vi "TaborBurst.vi"(0 "Input Cluster":T1={"Cycles"=0, "Therapy frequency (MHz)"=0.0, "Therapy amplitude (mV)"=50.0} {"Therapy amplitude (mV)" min=50.0 max=2000.0 format="%.2f"; "Therapy frequency (MHz)" format="%.2f"}, 1 "instrument in":refnum<k15>, 3 "error in (no error)":errorcluster) -> (5 "instrument out":refnum<k15>, 8 "error out":errorcluster)   [LabVIEW 2022 SP3]
uses:
  Pulsers/PulserGlobals.vi
panel:
  # "Set up to work with HP33120A. It is used as a burst source with\neither a gated burst or a fixed number of cycels"
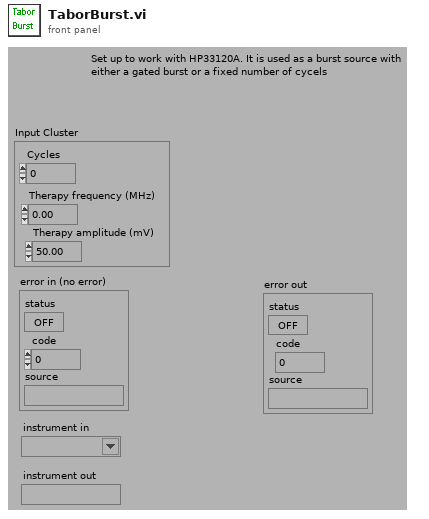
[diagram p1: front panel]
types:
  T1 = cluster{"Cycles":i32, "Therapy frequency (MHz)":dbl, "Therapy amplitude (mV)":dbl}
  T2 = cluster{"Therapy frequency (MHz)":dbl, "Therapy amplitude (mV)":dbl, "time therapy on (s)":dbl, "Therapy Delay (ms) ":dbl, "Time (s)":dbl}
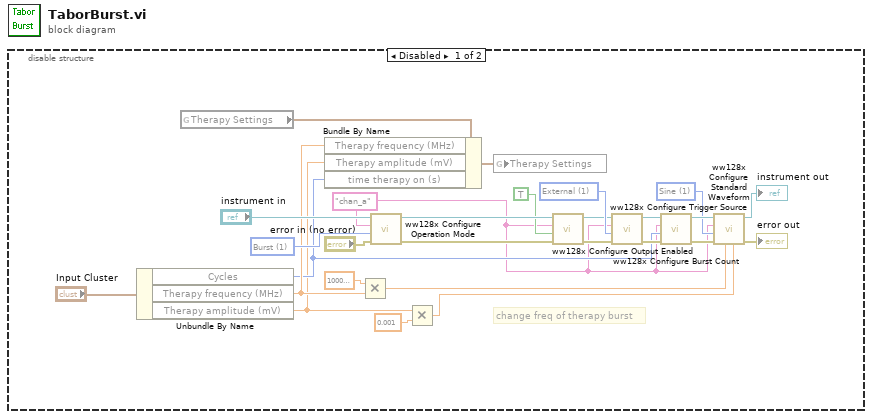
[diagram p0: block diagram]
diagram:
  n1 = disable-structure shown="Disabled" {
    frame Disabled {
      w1 = "chan_a" ("channel name (\"CHAN_A\")")
      w11 = 1 items=["External"=1, "Internal"=3, "Software Trigger"=2] ("source")
      w16 = 1 items=["Continuous"=0, "Burst"=1, "Gated"=1001, "Triggered"=1002] ("operation mode")
      w20 = 1 items=["Sine"=1, "Square"=2, "Triangle"=3, "Ramp Up"=4, "Ramp Down"=5, "DC"=6, "Ramp"=1001, "Pulse"=1005, "Sync"=1002, "Gaussian"=1003, "Exponential"=1004, "Noise"=1006] ("waveform")
      # "change freq of therapy burst"
      n2 = Unbundle By Name("Input Cluster") -> ("Cycles"=w3:i32, "Therapy frequency (MHz)"=w4:dbl, "Therapy amplitude (mV)"=w2:dbl)
      n3 = global read "PulserGlobals.vi" "Therapy Settings"() -> (w6:T2)
      n4 = Bundle By Name(cluster=w6, "Therapy frequency (MHz)"=w4, "Therapy amplitude (mV)"=w2, "time therapy on (s)"=w3) -> (w5:T2)
      n5 = Multiply(x=1000000.0, y=w4) -> (x*y=w21:dbl)
      n6 = call <instrlib>:"ww128x Configure Operation Mode.vi"("error in (no error)"="error in (no error)", "operation mode (Continuous)"=w16, "channel name (\"CHAN_A\")"=w1, "instrument handle"="instrument in") -> ("error out"=w13:errorcluster, "instrument handle out"=w15:refnum<k15>)  [unwired: 6 in]
      n7 = Multiply(x=w2, y=0.001) -> (x*y=w18:dbl)
      n8 = global write "PulserGlobals.vi" "Therapy Settings"(w5) -> ()
      n9 = call <instrlib>:"ww128x Configure Output Enabled.vi"("error in (no error)"=w13, "channel enabled (False)"=TRUE ("enabled"), "channel name (\"CHAN_A\")"=w1, "instrument handle"=w15) -> ("error out"=w9:errorcluster, "instrument handle out"=w10:refnum<k15>)  [unwired: 6 in]
      n10 = call <instrlib>:"ww128x Configure Trigger Source.vi"("error in (no error)"=w9, "trigger source (External)"=w11, "channel name (\"CHAN_A\")"=w1, "instrument handle"=w10) -> ("error out"=w7:errorcluster, "instrument handle out"=w8:refnum<k15>)  [unwired: 6 in]
      n11 = call <instrlib>:"ww128x Configure Burst Count.vi"("error in (no error)"=w7, "burst count (2)"=w3, "channel name (\"CHAN_A\")"=w1, "instrument handle"=w8) -> ("error out"=w25:errorcluster, "instrument handle out"=w26:refnum<k15>)  [unwired: 6 out]
      n12 = call <instrlib>:"ww128x Configure Standard Waveform.vi"("amplitude"=w18, "frequency"=w21, "error in (no error)"=w25, "waveform"=w20, "channel name"=w1, "instrument handle"=w26) -> ("error out"=→"error out":errorcluster, "instrument handle out"=→"instrument out":refnum<k15>)  [unwired: 2 in, 2 out]
    }
    frame Enabled {
    }
  }
